vi "4.7.3.vi"() -> ()   [LabVIEW 2017]
panel:
  out "Table":string[][](table)
  in  "OK Button":bool
  in  "stop":bool
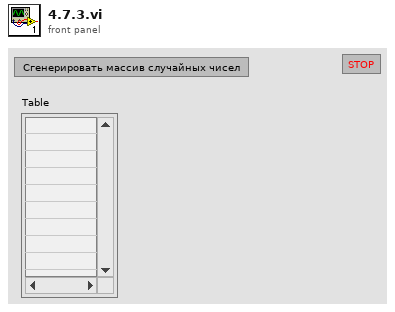
[diagram p1: front panel]
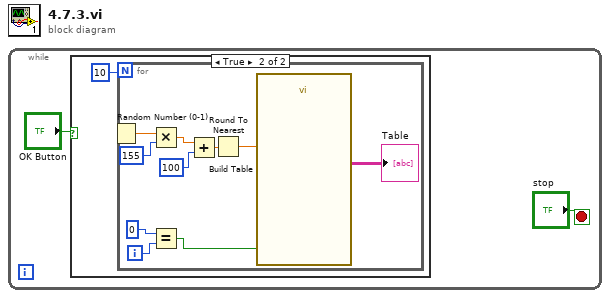
[diagram p0: block diagram]
diagram:
  n1 = while {
    stop <- "stop" stop-if-true
    n2 = case shown="True" "OK Button" {
      frame False {
      }
      frame True {
        n3 = for {
          N: 10 -> [_]
          i -> [w5]
          n4 = Random Number (0-1)() -> (number: 0 to 1=w12:dbl)
          n5 = Multiply(x=w12, y=155) -> (x*y=w13:dbl)
          n6 = Equal?(x=0, y=w5) -> (x = y?=w4:bool)
          n7 = Add(x=w13, y=100) -> (x+y=w11:dbl)
          n8 = Round To Nearest(number=w11) -> (nearest integer value=w7:dbl)
          n9 = call "Build Table"("Reset"=w4, "Signals"=w7) -> ("Table"=→"Table":string[][])  [unwired: 3 in, 6 out]
        }
      }
    }
  }
